vi "initial_check.vi"(1 "Data":dbl) -> (0 "String":string)   [LabVIEW 2017]
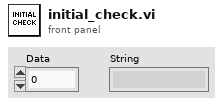
[diagram p1: front panel]
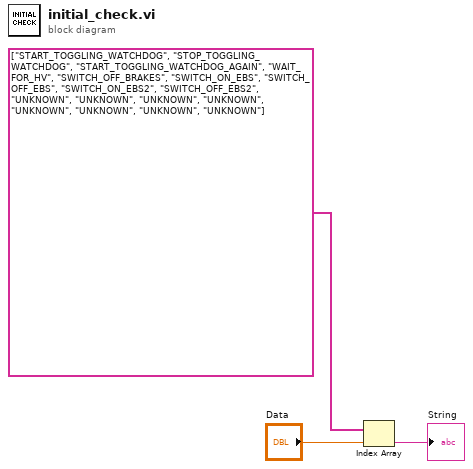
[diagram p0: block diagram]
diagram:
  n1 = Index Array(array=string[] ["START_TOGGLING_WATCHDOG", "STOP_TOGGLING_WATCHDOG", "START_TOGGLING_WATCHDOG_AGAIN", "WAIT_FOR_HV", "SWITCH_OFF_BRAKES", "SWITCH_ON_EBS", "SWITCH_OFF_EBS", "SWITCH_ON_EBS2", "SWITCH_OFF_EBS2", "UNKNOWN", "UNKNOWN", "UNKNOWN", "UNKNOWN", "UNKNOWN", "UNKNOWN", "UNKNOWN", "UNKNOWN"], index="Data") -> (element=→"String":string)
